vi "Update-motor-activity.vi"(8 "error in (no error)":errorcluster, 11 "Data in":T1) -> (0 "error out":errorcluster, 3 "Data out":T1)   [LabVIEW 2013, in "PowderDeposition.lvlib" / "PD-Main.lvclass"]
doc: "Activate the motors that are selected - correspondig button pressed - but not yet active."
uses:
  PD-Main.lvclass
  Object-reference.ctl
  PD-Main.lvclass/PD-Main.ctl
  Assembly/Motor-assembly.lvclass
  Motor/Motor.lvclass
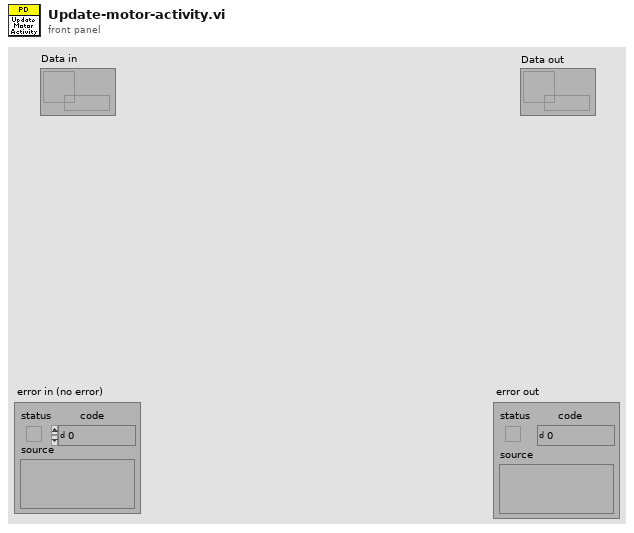
[diagram p1: front panel]
types:
  T1 = typedef "PowderDeposition.lvlib/PD-Main.lvclass/Object-reference.ctl" = refnum<data-value>
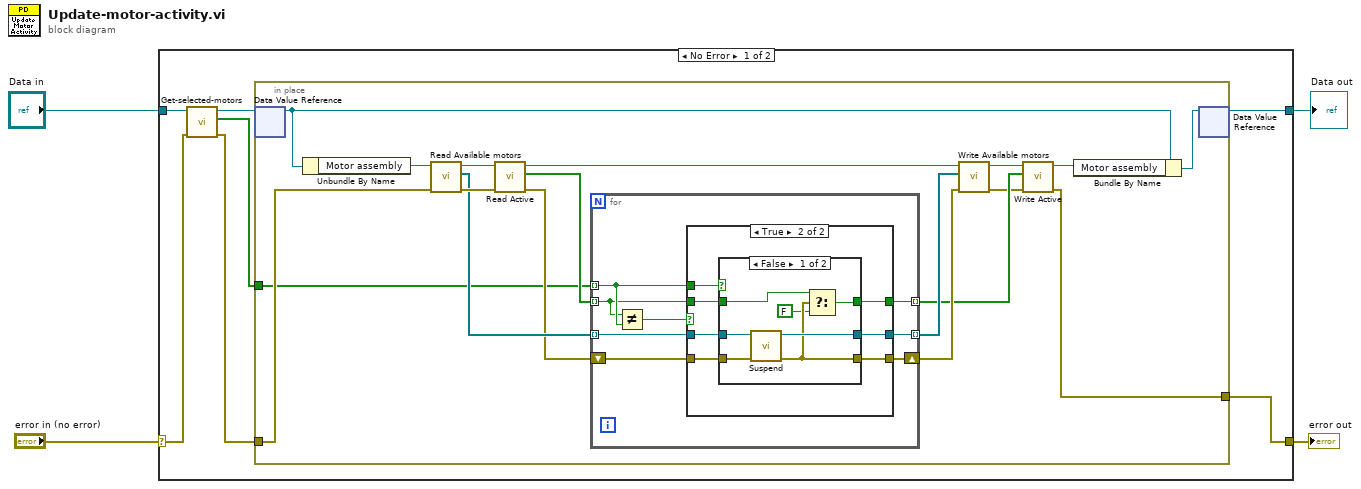
[diagram p0: block diagram]
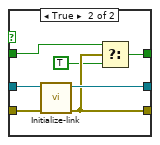
[diagram p3: hidden frame]
diagram:
  n1 = case shown="No Error" "error in (no error)" {
    selector: "error in (no error)" -> [w8 w63]
    tunnel: [w5 w63] -> w3
    tunnel: "Data in" -> [w11 w62]
    tunnel: [w10 w62] -> w1
    frame No Error {
      n2 = call "Get-selected-motors.vi"("error in (no error)"=w8, "Object ref in"=w11) -> ("error out"=w7:errorcluster, "Active?"=w6:bool[], "Object ref out"=w9:T1)  [unwired: 7 in]
      n3 = in-place {
        in-place-border: [w18] -> w5
        in-place-border: w7 -> [w17]
        in-place-border: w6 -> [w12]
        n4 = in-place-dvr #1(w9) -> (w14:refnum<class "PD-Main.lvclass">)  [unwired: 1 out]
        n5 = Unbundle By Name(w14) -> ("Motor assembly"=w16:refnum<class "Motor-assembly.lvclass">)
        n6 = call-dynamic "Read Available motors.vi"("error in (no error)"=w17, "Available motors in"=w16) -> ("error out"=w28:errorcluster, "Available motors"=w26:refnum<class "Motor.lvclass">[], "Available motors out"=w29:refnum<class "Motor-assembly.lvclass">)  [unwired: 7 in]
        n7 = call-dynamic "Read Active.vi"("error in (no error)"=w28, "Available motors in"=w29) -> ("error out"=w25:errorcluster, "Active?"=w27:bool[], "Available motors out"=w22:refnum<class "Motor-assembly.lvclass">)  [unwired: 7 in]
        n8 = for {
          tunnel: w12 -> [w31] mode=indexing
          tunnel: w27 -> [w30] mode=indexing
          tunnel: w26 -> [w37] mode=indexing
          tunnel: [w36] -> w23 mode=indexing
          shift-right: [w34] -> w24
          shift-left: w25 -> [w35]
          tunnel: [w33] -> w21 mode=indexing
          n9 = Not Equal?(x=w30, y=w31) -> (x != y?=w32:bool)
          n10 = case shown="True" w32 {
            tunnel: w31 -> [_ w47]
            tunnel: w37 -> [w39 w46]
            tunnel: [w39 w45] -> w36
            tunnel: w35 -> [w38 w44]
            tunnel: [w38 w43] -> w34
            tunnel: [w40 w42] -> w33
            tunnel: w30 -> [w40 w41]
            frame False {
            }
            frame True {
              n11 = case shown="False" w47 {
                tunnel: w46 -> [w54 w61]
                tunnel: [w52 w60] -> w45
                tunnel: w44 -> [w53 w59]
                tunnel: [w49 w57] -> w43
                tunnel: [w51 w58] -> w42
                tunnel: w41 -> [w50 w56]
                frame False {
                  n12 = call-dynamic "Suspend.vi"("error in (no error)"=w53, "Motor in"=w54) -> ("error out"=w49:errorcluster, "Motor out"=w52:refnum<class "Motor.lvclass">)  [unwired: 8 in]
                  n13 = Select(t=w50, s=w49, f=FALSE) -> (s? t:f=w51:bool)
                }
                frame True {
                  n14 = call-dynamic "Initialize-link.vi"("error in (no error)"=w59, "Motor in"=w61) -> ("error out"=w57:errorcluster, "Motor out"=w60:refnum<class "Motor.lvclass">)  [unwired: 8 in]
                  n15 = Select(t=w56, s=w57, f=TRUE) -> (s? t:f=w58:bool)
                }
              }
            }
          }
        }
        n16 = call-dynamic "Write Available motors.vi"("error in (no error)"=w24, "Available motors"=w23, "Available motors in"=w22) -> ("error out"=w19:errorcluster, "Available motors out"=w20:refnum<class "Motor-assembly.lvclass">)  [unwired: 7 in]
        n17 = call-dynamic "Write Active.vi"("error in (no error)"=w19, "Active?"=w21, "Available motors in"=w20) -> ("error out"=w18:errorcluster, "Available motors out"=w15:refnum<class "Motor-assembly.lvclass">)  [unwired: 7 in]
        n18 = Bundle By Name(cluster=w14, "Motor assembly"=w15) -> (w13:refnum<class "PD-Main.lvclass">)
        n19 = in-place-dvr #1(w13) -> (w10:T1)  [unwired: 1 out]
      }
    }
    frame Error {
    }
  }
  "error out" <- w3
  "Data out" <- w1
